vi "dataflow.vi"() -> ()   [LabVIEW 2017]
panel:
  in  "stop":bool
  in  "Boolean":bool
  out "Thermometer (C)":dbl(slide) scale=0.0..100.0
  in  "Temperature (F)":dbl(slide) scale=0.0..100.0
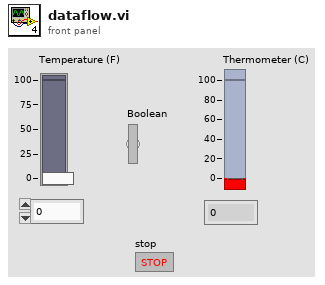
[diagram p1: front panel]
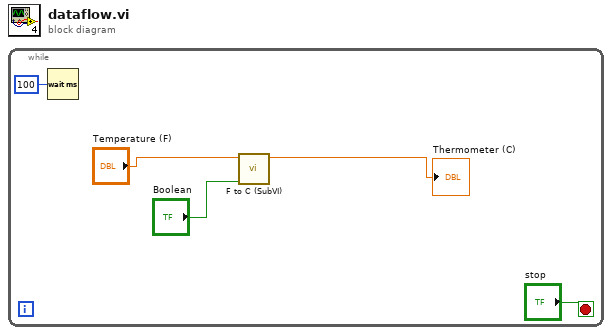
[diagram p0: block diagram]
diagram:
  n1 = while {
    stop <- "stop" stop-if-true
    n2 = Wait (ms)(milliseconds to wait=u32 100) -> ()  [unwired: 1 out]
    n3 = call "F to C (SubVI).vi"("Boolean"="Boolean", "Temperature (F)"="Temperature (F)") -> ("Numeric"=→"Thermometer (C)":dbl)  [unwired: 9 in]
  }
